vi "RunningAverage.GetResultChannelGroupData.vi"(8 "Error in":errorcluster, 9 "Enabled?":bool, 11 "Device Ref in":T1 format="%.0x") -> (0 "Error out":errorcluster, 2 "Group Data Array":T2(array[cluster]) {"VS Refs" format="%.0x"}, 3 "Device Ref out":T1=18446744073709551615 format="%.0x")   [LabVIEW 2015, in "Running Average.lvlib"]
uses:
  Running Average.lvlib
  <vilib>/NI Veristand/Custom Device API/Custom Device Item Ref.ctl
  Constants.vi
  <vilib>/NI Veristand/Custom Device API/Get Item Property (Dependent Node Pointer).vi
  System Explorer/Waveform-Processing-Custom-Device System Explorer.lvlib
  <vilib>/NI VeriStand/Custom Device API/Custom Device API.lvlib
  Waveform-Processing-Custom-Device Shared.lvlib
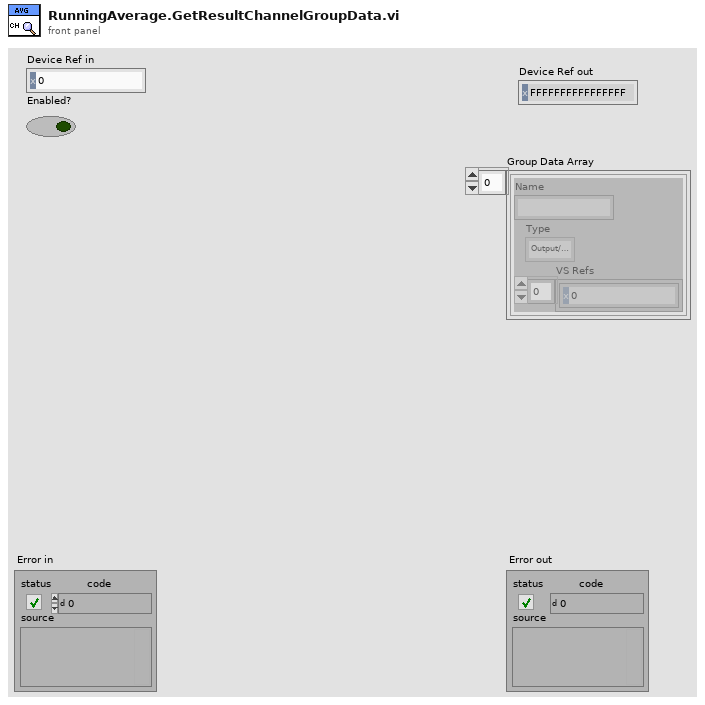
[diagram p1: front panel]
types:
  T1 = typedef "Custom Device API.lvlib/Custom Device Item Ref.ctl" = u64
  T2 = cluster{"Name":string, "Type":enum16{"Output/Write", "Input/Read", "Input/ReadWrite"}, "VS Refs":T1[]}[]
  T3 = enum16{"Output/Write", "Input/Read", "Input/ReadWrite"}
  T4 = cluster{"Name":string, "Type":enum16{"Output/Write", "Input/Read", "Input/ReadWrite"}, "VS Refs":T1[]}
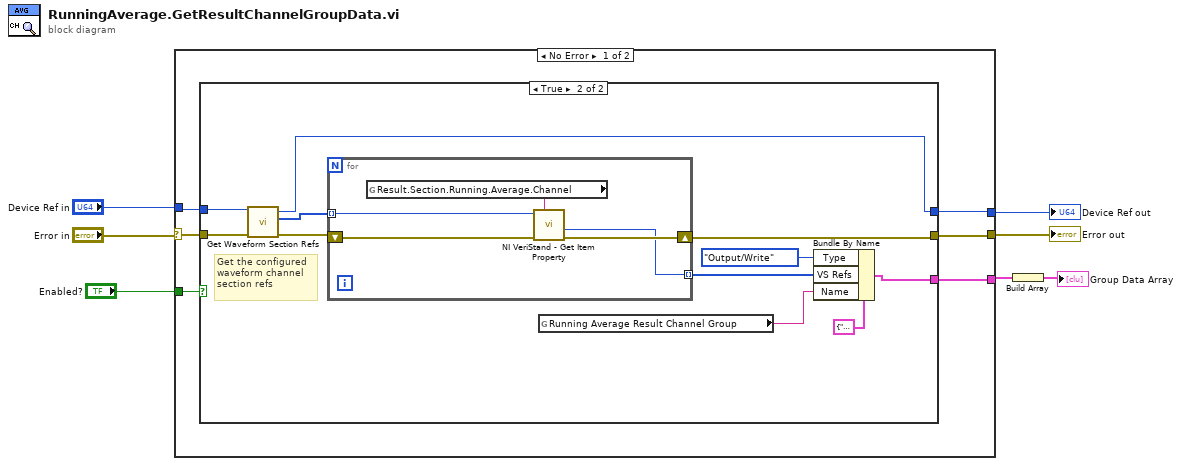
[diagram p0: block diagram]
diagram:
  n1 = case shown="No Error" "Error in" {
    selector: "Error in" -> [w13 w33]
    tunnel: [w11 w33] -> w6
    tunnel: "Device Ref in" -> [w12 w32]
    tunnel: "Enabled?" -> [w10 _]
    tunnel: [w9 w32] -> w3
    tunnel: [w8 _] -> w2
    frame No Error {
      n2 = case shown="True" w10 {
        tunnel: w13 -> [w15 w26]
        tunnel: w12 -> [w14 w24]
        tunnel: [w15 w17] -> w11
        tunnel: [w14 w16] -> w9
        tunnel: [_ w18] -> w8
        frame False {
        }
        frame True {
          # "Get the configured\nwaveform channel\nsection refs"
          n3 = call "Get Waveform Section Refs.vi"("Error in"=w26, "Device Ref in"=w24) -> ("Error out"=w25:errorcluster, "Result Section Refs"=w23:T1[], "Device Ref out"=w16:T1)  [unwired: 7 in]
          n4 = for {
            tunnel: w23 -> [w27] mode=indexing
            shift-right: [w29] -> w17
            shift-left: w25 -> [w31]
            tunnel: [w28] -> w22 mode=indexing
            n5 = global read "Constants.vi" "Result.Section.Running.Average.Channel"() -> (w30:string)
            n6 = call-poly <vilib>:"NI VeriStand - Get Item Property.vi"("error in (no error)"=w31, "Property Name"=w30, "Item Ref in"=w27) -> ("error out"=w29:errorcluster, "Dependent Node Ref"=w28:T1)  [unwired: 5 in, 2 out]
          }
          n7 = global read "Constants.vi" "Running Average Result Channel Group"() -> (w21:string)
          n8 = Bundle By Name(cluster=T4 {"Name"="", "Type"=enum."Output/Write", "VS Refs"=[]} ("Group"), "Type"=T3."Output/Write", "VS Refs"=w22, "Name"=w21) -> (w18:T4)
        }
      }
    }
    frame Error {
    }
  }
  "Error out" <- w6
  "Device Ref out" <- w3
  n9 = Build Array(w2) -> (→"Group Data Array":T2)
